vi "init.vi"() -> (2 "error out":errorcluster, 3 "GetDeviceInterface":refnum<k7>)   [LabVIEW 2019]
panel:
  out "element":string
  out "Device moved":bool
  in  "xphyspecLib.IXPhySpec 2":refnum<k7>
  out "Error message":string
  out "Device detected":bool
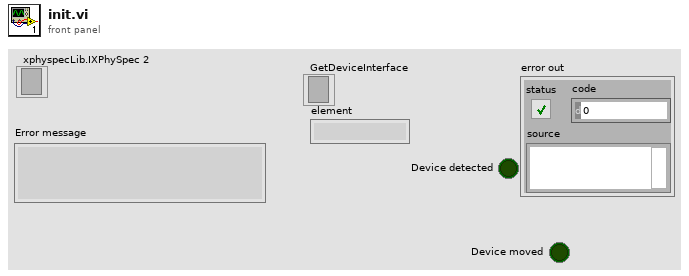
[diagram p1: front panel]
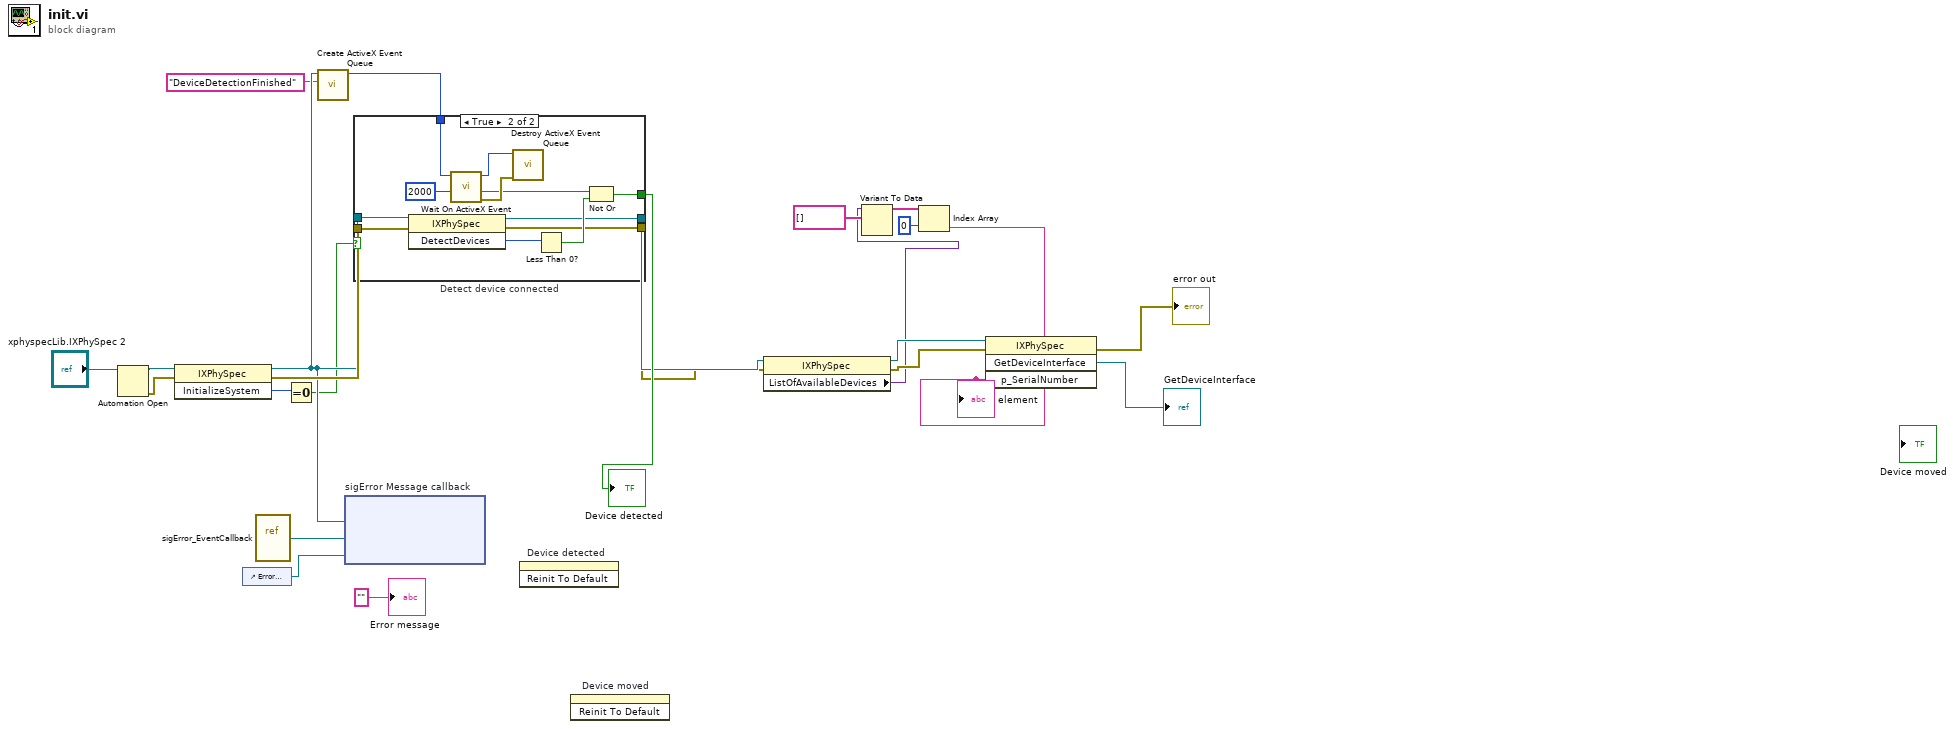
[diagram p0: block diagram]
diagram:
  n1 = Automation Open(Automation Refnum="xphyspecLib.IXPhySpec 2") -> (Automation Refnum=w13:refnum<k7>, error out=w14:errorcluster)  [unwired: 3 in]
  n2 = invoke class="IXPhySpec" method="InitializeSystem"(reference=w13, error in=w14) -> (reference out=w20:refnum<k7>, error out=w21:errorcluster, "InitializeSystem"=w15:i32)  [unwired: 1 in]
  n3 = control-ref of="Error message"() -> (w16:refnum<vi>)
  n4 = vi-ref "sigError_EventCallback.vi"() -> ("vi reference"=w17:refnum<vi>)
  n5 = Equal To 0?(x=w15) -> (x = 0?=w19:bool)
  n6 = call <vilib>:"Create ActiveX Event Queue.vi"("Event Name"="DeviceDetectionFinished", "Automation Refnum"=w20) -> ("Event Queue"=w22:i32)  [unwired: 4 in, 1 out]
  n7 = node "sigError Message callback"(w20, w17, w16) -> ()  [unwired: 2 in, 2 out]
  n8 = case "Detect device connected" shown="True" w19 {
    selector: w19 -> [w27 _]
    tunnel: w20 -> [w26 w39]
    tunnel: w21 -> [w25 w38]
    tunnel: w22 -> [_ w35]
    tunnel: [w26 w30] -> w11
    tunnel: [w25 w29] -> w10
    tunnel: [w27 w28] -> w23
    frame False {
    }
    frame True {
      n9 = invoke class="IXPhySpec" method="DetectDevices"(reference=w39, error in=w38) -> (reference out=w30:refnum<k7>, error out=w29:errorcluster, "DetectDevices"=w33:i32)  [unwired: 1 in]
      n10 = call <vilib>:"Wait On ActiveX Event.vi"("ms Timeout (-1)"=2000, "Event Queue"=w35) -> ("error out"=w34:errorcluster, "Timed Out"=w32:bool, "Event Queue Out"=w36:i32)  [unwired: 2 in, 1 out]
      n11 = call <vilib>:"Destroy ActiveX Event Queue.vi"("error in (no error)"=w34, "Event Queue"=w36) -> ()  [unwired: 5 in, 1 out]
      n12 = Less Than 0?(x=w33) -> (x < 0?=w31:bool)
      n13 = Not Or(1:w31, 2:w32) -> (0:w28:bool)
    }
  }
  "Device detected" <- w23
  n14 = invoke on="Device detected" class="Bool (strict)" method="Reinit To Default"() -> ()  [unwired: 3 in, 3 out]
  n15 = invoke on="Device moved" class="Bool (strict)" method="Reinit To Default"() -> ()  [unwired: 3 in, 3 out]
  n16 = property class="IXPhySpec"(reference=w11, error in=w10) -> (reference out=w9:refnum<k7>, error out=w8:errorcluster, "ListOfAvailableDevices"=w4:variant)
  n17 = Variant To Data(type=string[] [], Variant=w4) -> (data=w6:string[])  [unwired: 1 in, 1 out]
  n18 = Index Array(array=w6, index=0) -> (element=w3:string)
  "element" <- w3
  n19 = invoke class="IXPhySpec" method="GetDeviceInterface"(reference=w9, error in=w8, "p_SerialNumber"=w3) -> (error out=→"error out":errorcluster, "GetDeviceInterface"=→"GetDeviceInterface":refnum<k7>)  [unwired: 1 in, 2 out]
  "Error message" <- "" ("Error message")
